vi "ReadRaw.vi"() -> ()   [LabVIEW 2015]
uses:
  <vilib>/FPGAPlugInAG/USB-7855R OEM/niLvFpga_Open_USB-7855R OEM.vi
  <vilib>/rvi/interface/common/dynamic/niFpgaDynamicAddResources.vi
  <vilib>/Utility/error.llb/Error Cluster From Error Code.vi
  <vilib>/rvi/errors/niLvFpgaAdjustHostInterfaceError.vi
  <vilib>/measure/matone.llb/Extract Single Tone Information 1 Chan.vi
  <vilib>/FPGAPlugInAG/Dynamic/niLvFpga_Close_Dynamic.vi
  <vilib>/rvi/interface/nirviOpenFPGA/nirviOpenFPGA.xnode
  FPGA Bitfiles/DloopFunds_FPGATarget_SendRaw2_XaiqW2Sbois.lvbitx
  SendRaw.vi
  <vilib>/rvi/interface/nirviReadWriteControl/nirviReadWriteControl.xnode
  <vilib>/rvi/interface/nirviMethod/nirviMethod.xnode
  <vilib>/rvi/interface/nirviCloseFPGA/nirviCloseFPGA.xnode
  <vilib>/Analysis/NI_AALPro.lvlib
  <vilib>/measure/NI_MAPro.lvlib
  NiFpgaLv.dll
  <vilib>/rvi/interface/Simulation/niFpgaSimulationCallBeginRW.vi
  <vilib>/FPGAPlugInAG/Dynamic/niLvFpga_ReadFifo_Dynamic.vi
  <vilib>/rvi/errors/niLvFpgaMergeErrorWithErrorCode.vi
panel:
  out "Signal 3":waveform(dbl)(graph)
  in  "Input Period (ticks) 3":i16=80
  in  "Stop at peak 3":bool
  in  "Peak height 3":fxp<+/-,16,4>
  out "Output time 3":dbl
  out "Frequ 3":dbl
  out "Signal 2":waveform(dbl)(graph)
  in  "Input Period (ticks) 2":i16=80
  in  "Stop at peak 2":bool
  in  "Peak height 2":fxp<+/-,16,4>
  out "Output time 2":dbl
  out "Frequ 2":dbl
  out "Frequ":dbl
  out "Output time":dbl
  in  "Peak height":fxp<+/-,16,4>
  in  "Stop at peak":bool
  in  "Input Period (ticks)":i16=80
  out "Signal":waveform(dbl)(graph)
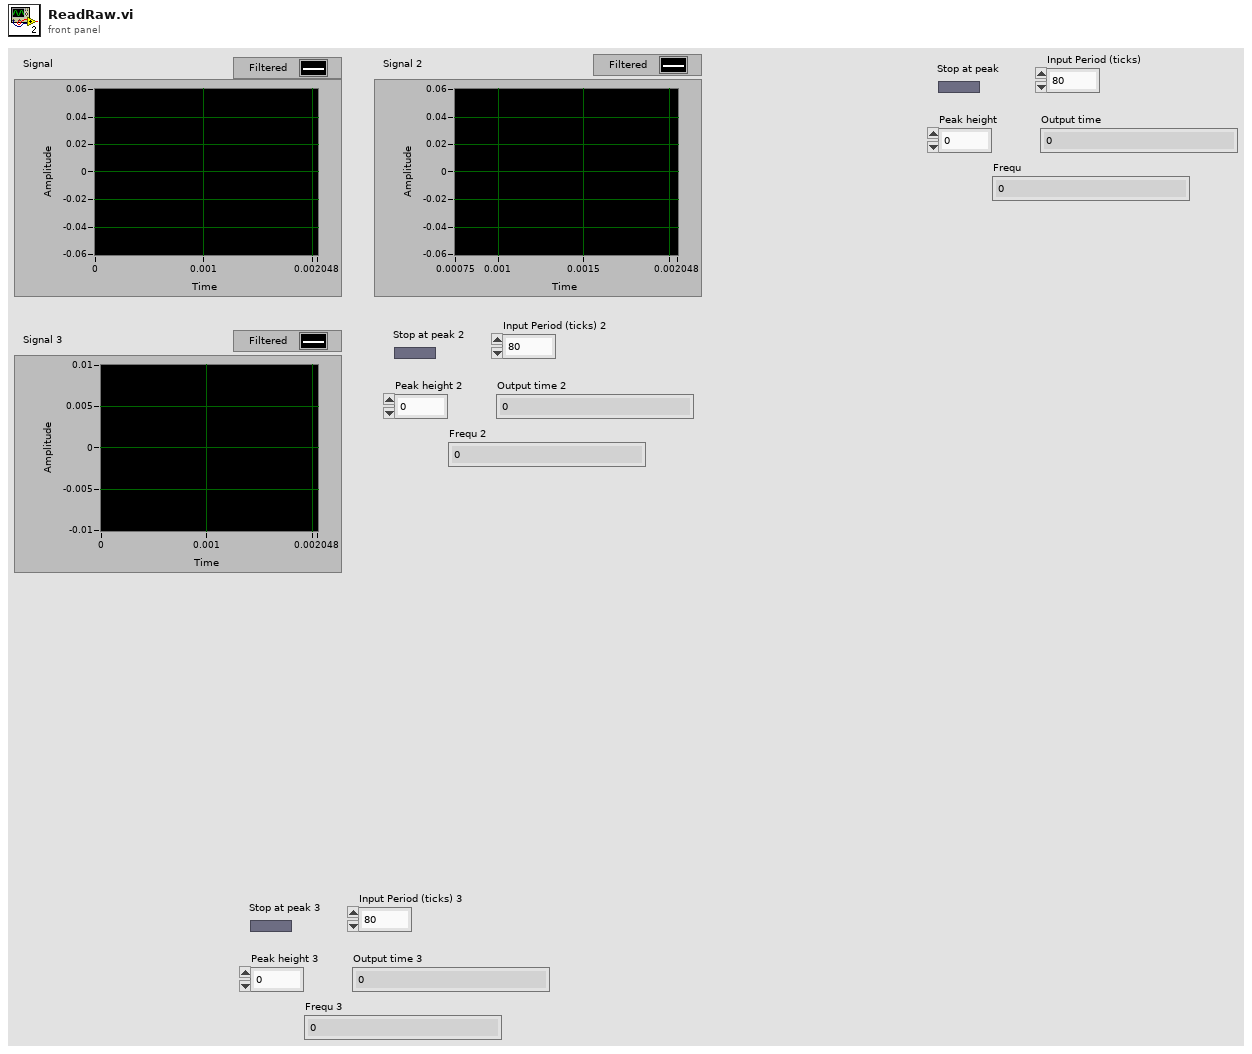
[diagram p1: front panel]
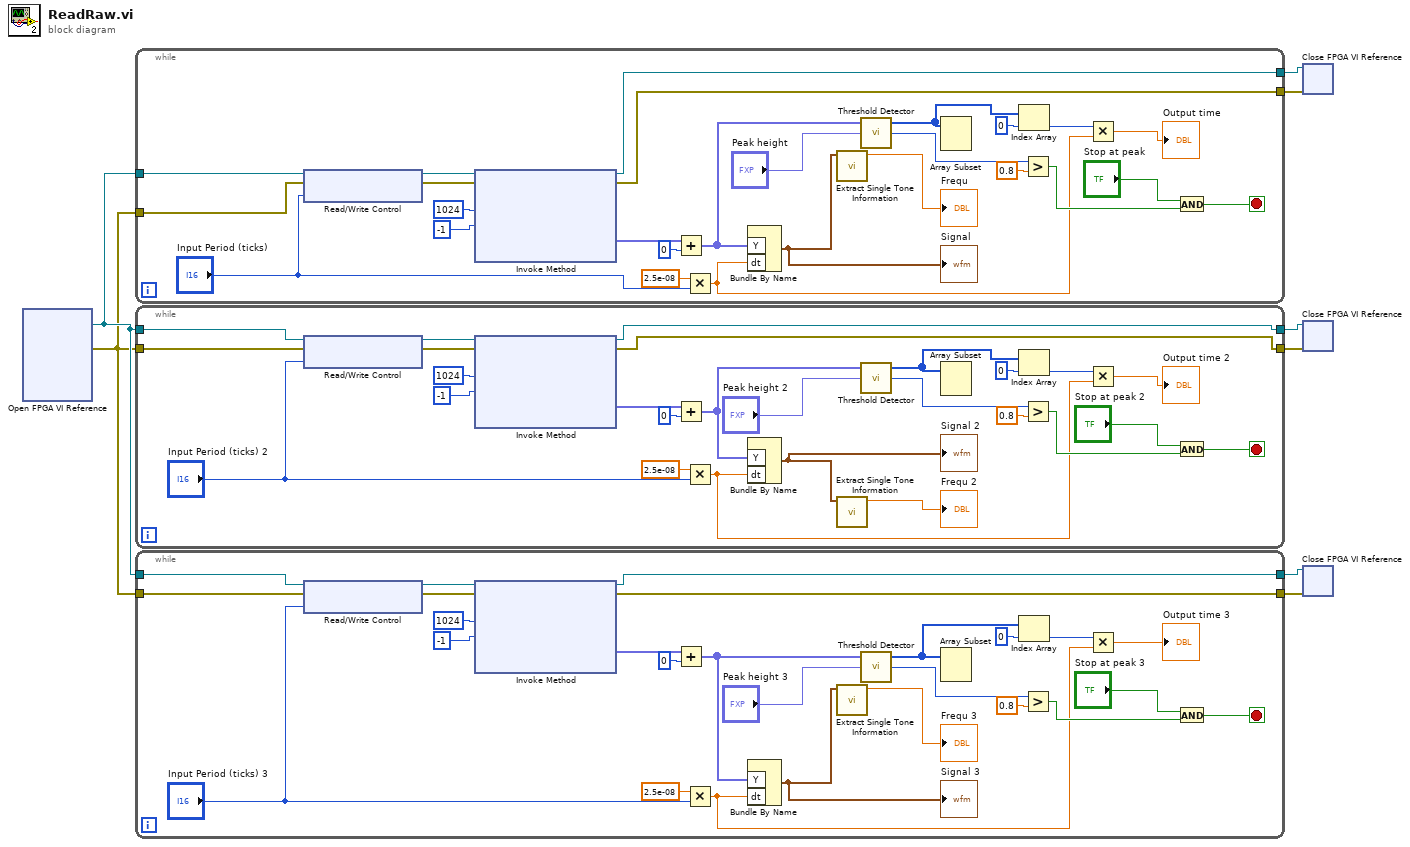
[diagram p0: block diagram]
diagram:
  n1 = xnode "Open FPGA VI Reference"() -> ("FPGA VI Reference Out"=w2:refnum<k20>, "error out"=w1:errorcluster)  [unwired: 2 in]
  n2 = while {
    tunnel: [w27] -> w8
    tunnel: [w33] -> w7
    tunnel: w2 -> [w31]
    tunnel: w1 -> [w30]
    stop <- w25 stop-if-true
    n3 = xnode "Read/Write Control"("FPGA VI Reference In"=w31, "error in"=w30, "Input period (ticks)"="Input Period (ticks)") -> ("FPGA VI Reference Out"=w28:refnum<k20>, "error out"=w29:errorcluster)
    n4 = xnode "Invoke Method"("FPGA VI Reference In"=w28, "error in"=w29, "Number of Elements"=1024, "Timeout (ms)"=-1) -> ("FPGA VI Reference Out"=w27:refnum<k20>, "error out"=w33:errorcluster, "Data"=w15:fxp<+/-,32,16>[])  [unwired: 1 out]
    n5 = Add(x=w15, y=0) -> (x+y=w14:fxp<+/-,49,33>[])
    n6 = Multiply(x=2.5e-08, y="Input Period (ticks)") -> (x*y=w17:dbl)
    n7 = Bundle By Name("Y"=w14, "dt"=w17) -> (w9:waveform(dbl))  [unwired: 1 in]
    "Signal" <- w9
    n8 = call-poly <vilib>:"Extract Single Tone Information.vi"("time signal in"=w9) -> ("detected frequency"=→"Frequ":dbl)  [unwired: 5 in, 5 out]
    n9 = call <vilib>:"Threshold Detector.vi"("threshold"="Peak height", "X"=w14) -> ("count"=w22:i32, "Indices"=w11:i32[])  [unwired: 1 in, 1 out]
    n10 = Array Subset(array=w11) -> ()  [unwired: 2 in, 1 out]
    n11 = Index Array(array=w11, index=0) -> (element=w18:i32)
    n12 = Greater?(x=w22, y=0.8) -> (0:w20:bool)
    n13 = Multiply(x=w18, y=w17) -> (x*y=→"Output time":dbl)
    n14 = And(x="Stop at peak", y=w20) -> (x .and. y?=w25:bool)
  }
  n15 = while {
    tunnel: [w53] -> w6
    tunnel: [w59] -> w5
    tunnel: w2 -> [w57]
    tunnel: w1 -> [w56]
    stop <- w51 stop-if-true
    n16 = xnode "Read/Write Control"("FPGA VI Reference In"=w57, "error in"=w56, "Input period (ticks)"="Input Period (ticks) 2") -> ("FPGA VI Reference Out"=w54:refnum<k20>, "error out"=w55:errorcluster)
    n17 = xnode "Invoke Method"("FPGA VI Reference In"=w54, "error in"=w55, "Number of Elements"=1024, "Timeout (ms)"=-1) -> ("FPGA VI Reference Out"=w53:refnum<k20>, "error out"=w59:errorcluster, "Data"=w41:fxp<+/-,32,16>[])  [unwired: 1 out]
    n18 = Add(x=w41, y=0) -> (x+y=w40:fxp<+/-,49,33>[])
    n19 = Multiply(x=2.5e-08, y="Input Period (ticks) 2") -> (x*y=w43:dbl)
    n20 = Bundle By Name("Y"=w40, "dt"=w43) -> (w35:waveform(dbl))  [unwired: 1 in]
    "Signal 2" <- w35
    n21 = call-poly <vilib>:"Extract Single Tone Information.vi"("time signal in"=w35) -> ("detected frequency"=→"Frequ 2":dbl)  [unwired: 5 in, 5 out]
    n22 = call <vilib>:"Threshold Detector.vi"("threshold"="Peak height 2", "X"=w40) -> ("count"=w48:i32, "Indices"=w37:i32[])  [unwired: 1 in, 1 out]
    n23 = Array Subset(array=w37) -> ()  [unwired: 2 in, 1 out]
    n24 = Index Array(array=w37, index=0) -> (element=w44:i32)
    n25 = Greater?(x=w48, y=0.8) -> (0:w46:bool)
    n26 = Multiply(x=w44, y=w43) -> (x*y=→"Output time 2":dbl)
    n27 = And(x="Stop at peak 2", y=w46) -> (x .and. y?=w51:bool)
  }
  n28 = while {
    tunnel: [w79] -> w4
    tunnel: [w85] -> w3
    tunnel: w2 -> [w83]
    tunnel: w1 -> [w82]
    stop <- w77 stop-if-true
    n29 = xnode "Read/Write Control"("FPGA VI Reference In"=w83, "error in"=w82, "Input period (ticks)"="Input Period (ticks) 3") -> ("FPGA VI Reference Out"=w80:refnum<k20>, "error out"=w81:errorcluster)
    n30 = xnode "Invoke Method"("FPGA VI Reference In"=w80, "error in"=w81, "Number of Elements"=1024, "Timeout (ms)"=-1) -> ("FPGA VI Reference Out"=w79:refnum<k20>, "error out"=w85:errorcluster, "Data"=w67:fxp<+/-,32,16>[])  [unwired: 1 out]
    n31 = Add(x=w67, y=0) -> (x+y=w66:fxp<+/-,49,33>[])
    n32 = Multiply(x=2.5e-08, y="Input Period (ticks) 3") -> (x*y=w69:dbl)
    n33 = Bundle By Name("Y"=w66, "dt"=w69) -> (w61:waveform(dbl))  [unwired: 1 in]
    "Signal 3" <- w61
    n34 = call-poly <vilib>:"Extract Single Tone Information.vi"("time signal in"=w61) -> ("detected frequency"=→"Frequ 3":dbl)  [unwired: 5 in, 5 out]
    n35 = call <vilib>:"Threshold Detector.vi"("threshold"="Peak height 3", "X"=w66) -> ("count"=w74:i32, "Indices"=w63:i32[])  [unwired: 1 in, 1 out]
    n36 = Array Subset(array=w63) -> ()  [unwired: 2 in, 1 out]
    n37 = Index Array(array=w63, index=0) -> (element=w70:i32)
    n38 = Greater?(x=w74, y=0.8) -> (0:w72:bool)
    n39 = Multiply(x=w70, y=w69) -> (x*y=→"Output time 3":dbl)
    n40 = And(x="Stop at peak 3", y=w72) -> (x .and. y?=w77:bool)
  }
  n41 = xnode "Close FPGA VI Reference"("FPGA VI Reference In"=w8, "error in"=w7) -> ()  [unwired: 1 out]
  n42 = xnode "Close FPGA VI Reference"("FPGA VI Reference In"=w6, "error in"=w5) -> ()  [unwired: 1 out]
  n43 = xnode "Close FPGA VI Reference"("FPGA VI Reference In"=w4, "error in"=w3) -> ()  [unwired: 1 out]
